vi "AB_User_Log_Errors.vi"(8 "error in (no error)":errorcluster) -> (0 "error out":errorcluster)   [LabVIEW 2020]
uses:
  <vilib>/AppBuilder/logging/AB_Log_File_Action.ctl
  <resource>/Framework/Providers/Common/provcom_StringGlobals.vi
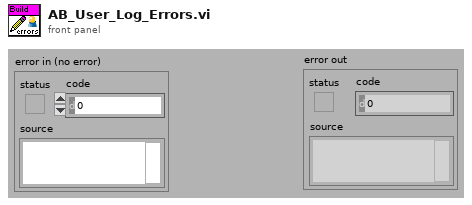
[diagram p1: front panel]
types:
  T1 = typedef "AB_Log_File_Action.ctl" = enum16{"write", "open", "close"}
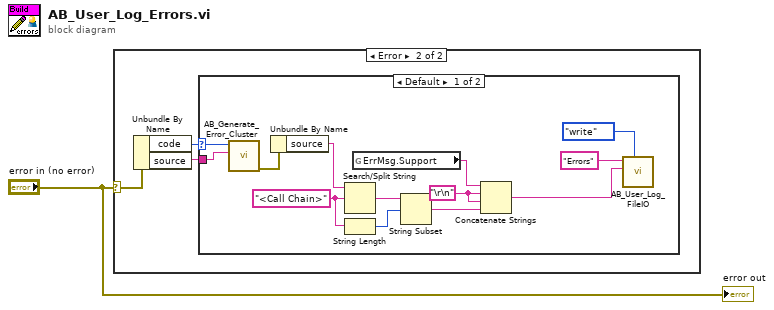
[diagram p0: block diagram]
diagram:
  n1 = case shown="Error" "error in (no error)" {
    selector: "error in (no error)" -> [_ w2]
    frame No Error {
    }
    frame Error {
      n2 = Unbundle By Name(w2) -> ("code"=w4:i32, "source"=w3:string)
      n3 = case shown="Default" w4 {
        selector: w4 -> [w14 _]
        tunnel: w3 -> [w13 _]
        frame Default {
          w7 = "\r\n"
          w11 = "<Call Chain>" ("search string/char (-)")
          n4 = call <vilib>:"AB_Generate_Error_Cluster.vi"("source"=w13, "Code"=w14) -> ("error out"=w15:errorcluster)  [unwired: 9 in]
          n5 = Unbundle By Name(w15) -> ("source"=w6:string)
          n6 = Search/Split String(string=w6, search string/char (-)=w11) -> (match + rest of string=w10:string)  [unwired: 3 out]
          n7 = String Length(string=w11) -> (length=w9:i32)
          n8 = global read "provcom_StringGlobals.vi" "ErrMsg.Support"() -> (w12:string)
          n9 = String Subset(string=w10, offset (0)=w9) -> (substring=w8:string)  [unwired: 1 out]
          n10 = Concatenate Strings(w12, w7, w7, w8) -> (w5:string)
          n11 = call <vilib>:"AB_User_Log_FileIO.vi"("fileAction"=AB_Log_File_Action."write", "data"=w5, "newSection"="Errors") -> ()  [unwired: 2 in, 7 out]
        }
        frame 43 {
          # "User cancelling is not an error."
        }
      }
    }
  }
  "error out" <- "error in (no error)"
